vi "Shutdown.vi"(8 "error in":errorcluster, 11 "Control Box in":refnum<class "Control Box.lvclass">) -> (0 "error out":errorcluster, 3 "Control Box out":refnum<class "Control Box.lvclass">)   [LabVIEW 2018, in "Control Box.lvlib" / "Control Box.lvclass"]
uses:
  Control Box.lvclass
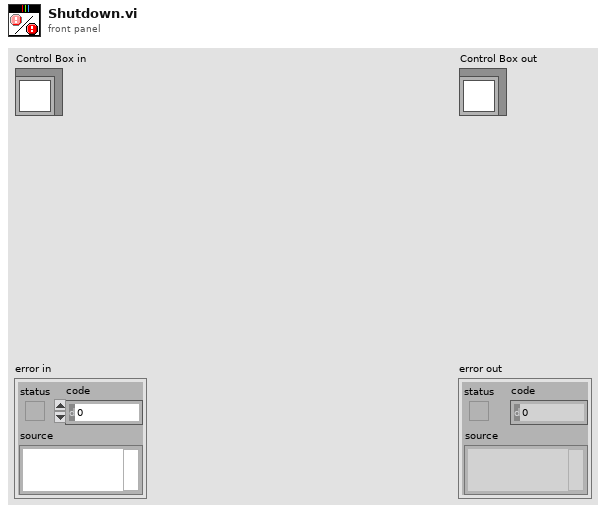
[diagram p1: front panel]
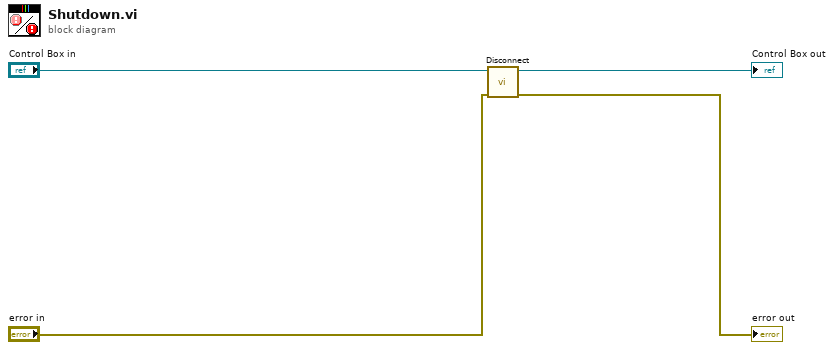
[diagram p0: block diagram]
diagram:
  n1 = call-dynamic "Disconnect.vi"("error in"="error in", "Control Box in"="Control Box in") -> ("error out"=→"error out":errorcluster, "Control Box out"=→"Control Box out":refnum<class "Control Box.lvclass">)  [unwired: 8 in]
